vi "Set I2 (SubVI).vi"(11 "Current Y":string) -> (3 "String":string)   [LabVIEW 2018]
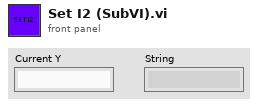
[diagram p1: front panel]
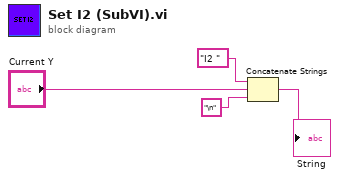
[diagram p0: block diagram]
diagram:
  n1 = Concatenate Strings("I2 ", "Current Y", "\n") -> (→"String":string)
